vi "LVClass_ComputePhaseSet GetZonalPrefs.vi"(0 "ComputePhaseSet in":refnum<class "ComputePhaseSet.lvclass">, 11 "error in (no error)":errorcluster) -> (4 "ComputePhaseSet out":refnum<class "ComputePhaseSet.lvclass">, 6 "WavefrontSetup.ZonalSetup":T1={"Number of weak iterations"=6, "Number of max iterations"=100, "Residual limit"=5e-05}, 15 "error out":errorcluster)   [LabVIEW 2020, in "ComputePhaseSet.lvclass"]
doc: "Get preferences for zonal phase reconstruction.\n\n--------------------------------------------------------------------------------\n\n<B>ComputePhaseSetIn </B> : ComputePhaseSet object.\n<B>ComputePhaseSetOut </B> : ComputePhaseSet object.\n<B>nb_weak_iterations </B> : Maximum number of weak iterations. A weak iteration is defined as an iteration\n for which the variation of the residue from previous iteration is below the\n residual_limit multiplied by the number of microlenses of the Haso.\n<B>nb_max_iterations </B> : Maximum number of iterations.\n<B>residual_limit </B> : Residual variation limit.\n<B>ErrorIn </B> : Error\n<B>ErrorOut </B> : Error\n\n--------------------------------------------------------------------------------"
uses:
  ComputePhaseSet.lvclass
  ZonalPrefs.ctl
  ComputePhaseSet.lvclass/ComputePhaseSet.ctl
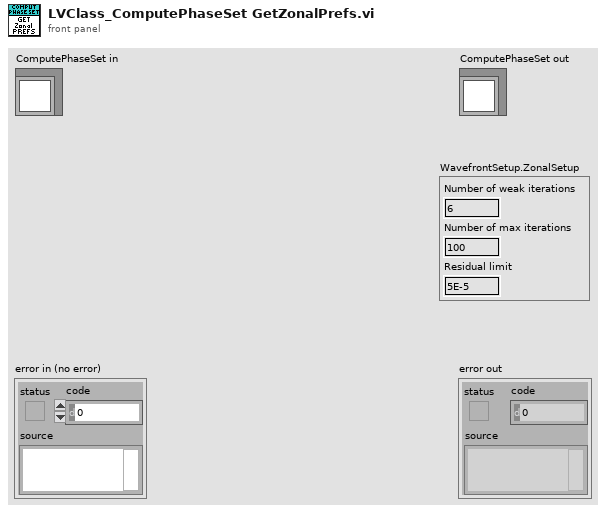
[diagram p1: front panel]
types:
  T1 = typedef "ZonalPrefs.ctl" = cluster{"Number of weak iterations":u16, "Number of max iterations":u32, "Residual limit":sgl}
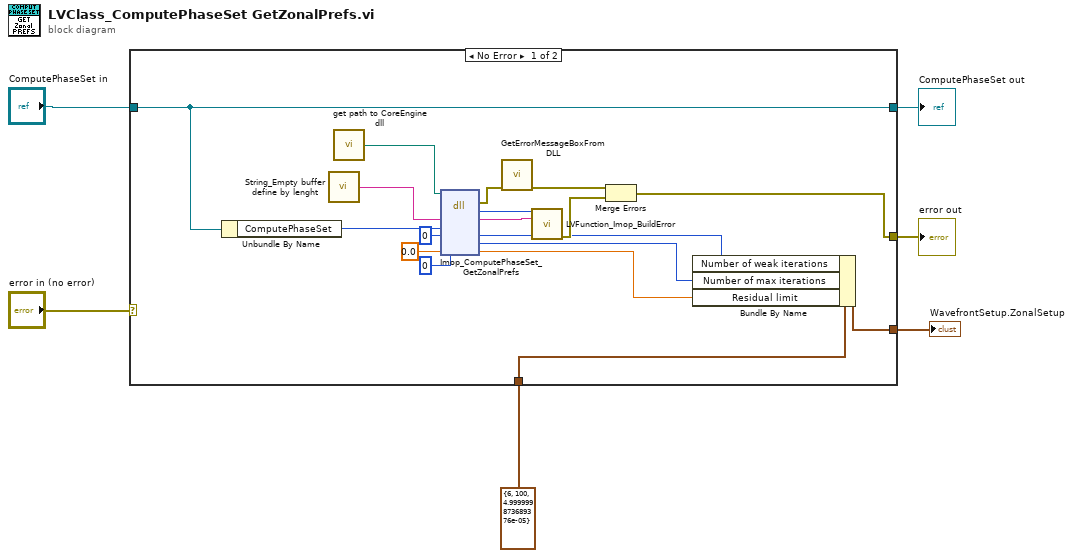
[diagram p0: block diagram]
diagram:
  n1 = case shown="No Error" "error in (no error)" {
    selector: "error in (no error)" -> [_ w27]
    tunnel: [w12 w27] -> w3
    tunnel: [w16 w26] -> w5
    tunnel: "ComputePhaseSet in" -> [w16 w26]
    tunnel: [w7 w25] -> w2
    tunnel: T1 {"Number of weak iterations"=6, "Number of max iterations"=100, "Residual limit"=5e-05} ("WavefrontSetup.ZonalSetup") -> [w11 w25]
    frame No Error {
      n2 = Unbundle By Name(w16) -> ("ComputePhaseSet"=w15:i32)
      n3 = call "String_Empty buffer define by lenght.vi"() -> ("Empty buffer"=w22:string)  [unwired: 1 in]
      n4 = call "get path to CoreEngine dll.vi"() -> ("path to c_interface_vc100.dll"=w21:path)  [unwired: 12 in, 3 out]
      n5 = dll-call lib="D:/2_trunk/Soft_haso/ImOpCoreEngine4_LV2011/DLLs/ImopEngine4_vc100.dll" fn="Imop_ComputePhaseSet_GetZonalPrefs"(path in=w21, "message"=w22, "objet"=w15, "nb_weak_iterations"=u32 0, "nb_max_iterations"=u32 0, "residual_limit"=sgl 0.0) -> (error out=w20:errorcluster, "return type"=w24:i32, "message"=w23:string, "nb_weak_iterations"=w10:u32, "nb_max_iterations"=w9:u32, "residual_limit"=w8:sgl)  [unwired: 3 in, 1 out]
      n6 = call "GetErrorMessageBoxFromDLL.vi"("error IN"=w20) -> ("error OUT"=w14:errorcluster)  [unwired: 10 in]
      n7 = call "LVFunction_Imop_BuildError.vi"("code"=w24, "String to Prepend to source (\"\")"=w23) -> ("error out"=w13:errorcluster)  [unwired: 13 in]
      n8 = Merge Errors(w14, w13) -> (w12:errorcluster)
      n9 = Bundle By Name(cluster=w11, "Number of weak iterations"=w10, "Number of max iterations"=w9, "Residual limit"=w8) -> (w7:T1)
    }
    frame Error {
    }
  }
  "error out" <- w3
  "ComputePhaseSet out" <- w5
  "WavefrontSetup.ZonalSetup" <- w2
